vi "Ctor.vi"(8 "error in (no error)":errorcluster, 11 "BluePlotHandle in":refnum<class "NIringPlotHandle.lvclass">) -> (0 "error out":errorcluster, 3 "BluePlotHandle out":refnum<class "NIringPlotHandle.lvclass">)   [LabVIEW 2021, in "NIringPlotHandle.lvclass"]
uses:
  NIringPlotHandle.lvclass
  NIringPlotHandle.lvclass/NIringPlotHandle.ctl
  RocketPlotHandle/RocketPlotHandle.lvclass
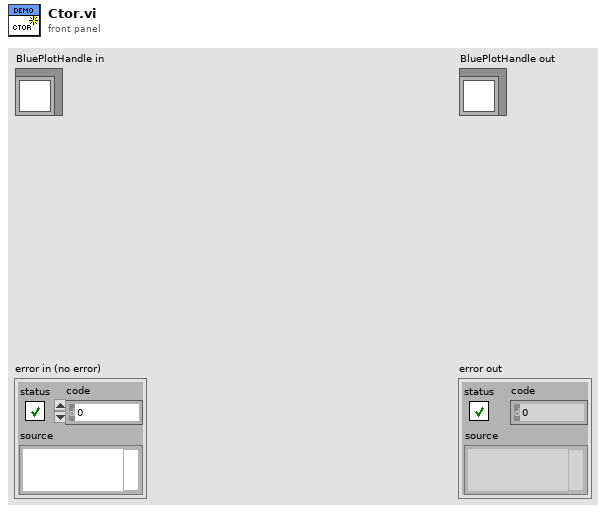
[diagram p1: front panel]
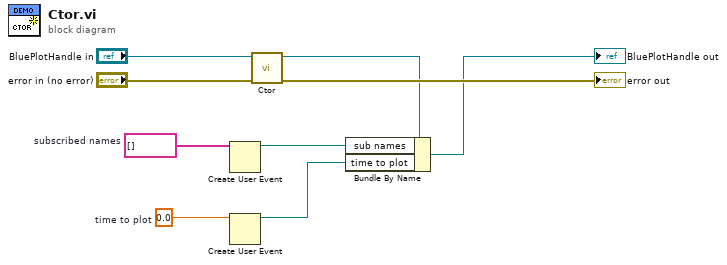
[diagram p0: block diagram]
diagram:
  w5 = 0.0  # time to plot
  w6 = string[] []  # subscribed names
  n1 = Create User Event(user event datatype=w6) -> (user event=w3:refnum<user-event>)  [unwired: 1 in, 1 out]
  n2 = Create User Event(user event datatype=w5) -> (user event=w2:refnum<user-event>)  [unwired: 1 in, 1 out]
  n3 = call-parent "Ctor.vi"("error in (no error)"="error in (no error)", "BluePlotHandle in"="BluePlotHandle in") -> ("error out"=→"error out":errorcluster, "BluePlotHandle out"=w4:refnum<class "NIringPlotHandle.lvclass">)  [unwired: 8 in]
  n4 = Bundle By Name(cluster=w4, "sub names"=w3, "time to plot"=w2) -> (→"BluePlotHandle out":refnum<class "NIringPlotHandle.lvclass">)
